vi "Handle WOTMotor Speeds.vi"(1 "Take in ball":bool, 2 "Bring in WOT":bool, 3 "Push out ball":bool) -> (0 "Wheels on Top":dbl)   [LabVIEW 2013]
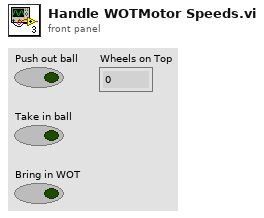
[diagram p1: front panel]
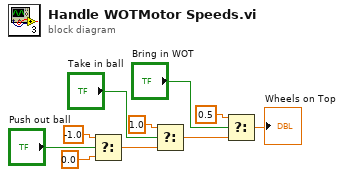
[diagram p0: block diagram]
diagram:
  n1 = Select(t=-1.0, s="Push out ball", f=0.0 ("t")) -> (s? t:f=w4:dbl)
  n2 = Select(t=1.0, s="Take in ball", f=w4) -> (s? t:f=w5:dbl)
  n3 = Select(t=0.5, s="Bring in WOT", f=w5) -> (s? t:f=→"Wheels on Top":dbl)
